vi "Key - MCListbox Read.vi"(8 "error in (no error)":errorcluster, 9 "New MulticolumnListbox Ref":refnum<vi>, 10 "Original MulticolumnListbox Ref":refnum<vi>, 11 "refnum":T1) -> (0 "error out":errorcluster, 2 "size(s)":i32[](array[numeric]), 3 "Refnum out":T1, 5 "Column Header Strings[]":string[](array[string]))   [LabVIEW 2013]
uses:
  <vilib>/Utility/config.llb/Config Data RefNum.ctl
  <vilib>/Utility/config.llb/Read Key (String).vi
  <vilib>/Utility/config.llb/NI_LVConfig.lvlib
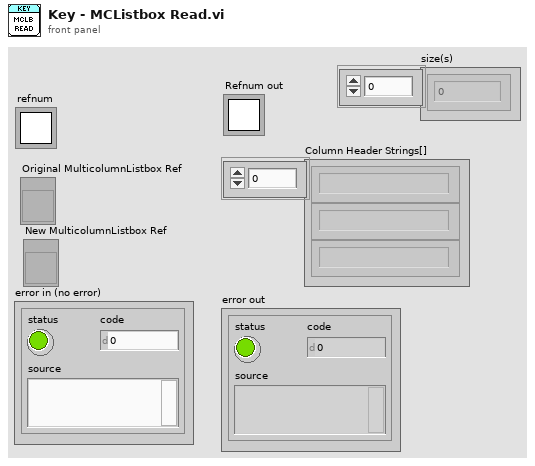
[diagram p1: front panel]
types:
  T1 = typedef "NI_LVConfig.lvlib/Config Data RefNum.ctl" = refnum<k1>
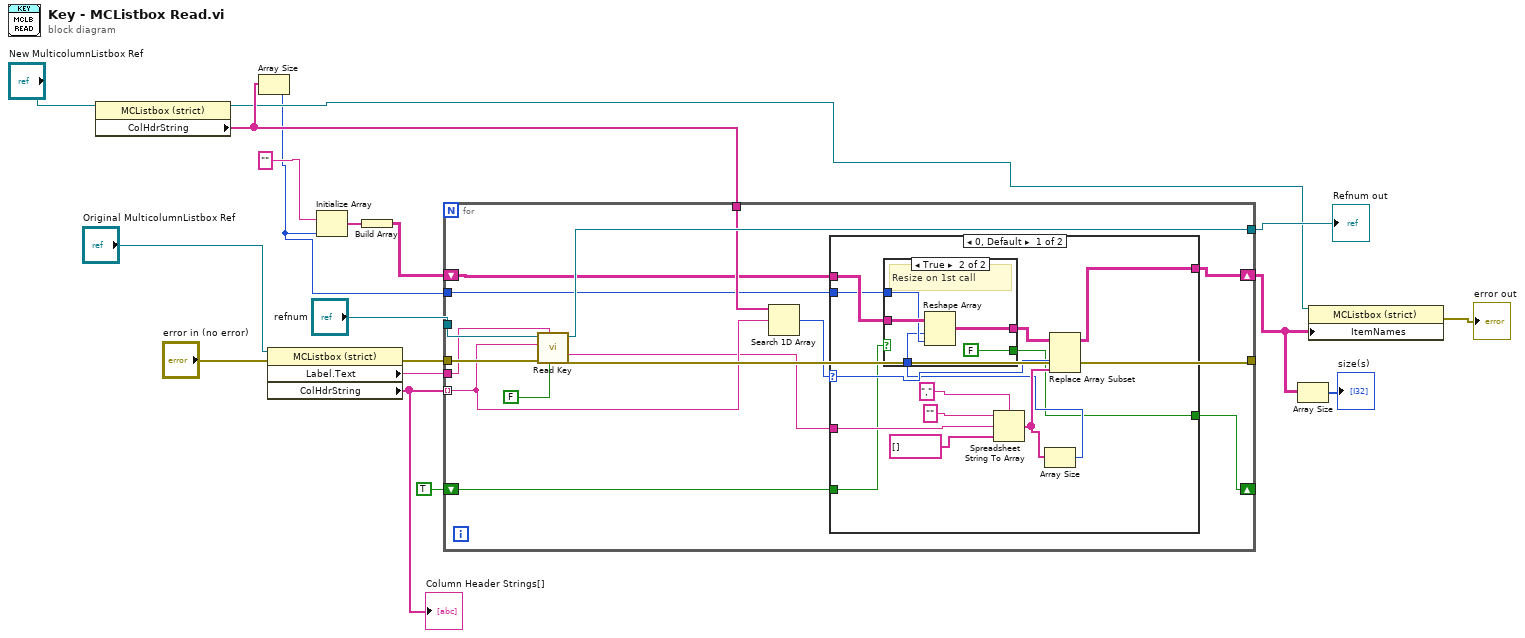
[diagram p0: block diagram]
diagram:
  n1 = property on="Property Node" class="MCListbox (strict)"(reference="New MulticolumnListbox Ref") -> (reference out=w10:refnum<vi>, "ColHdrString"=w11:string[])  [unwired: 1 in, 1 out]
  n2 = Array Size(array=w11) -> (size(s)=w5:i32)
  n3 = property on="Property Node" class="MCListbox (strict)"(reference="Original MulticolumnListbox Ref", error in="error in (no error)") -> (error out=w18:errorcluster, "Label.Text"=w13:string, "ColHdrString"=w4:string[])  [unwired: 1 out]
  "Column Header Strings[]" <- w4
  n4 = Initialize Array("" ("element"), w5) -> (w7:string[])
  n5 = Build Array(w7) -> (w6:string[][])
  n6 = for {
    tunnel: w18 -> [w33]
    tunnel: [w32] -> _
    tunnel: [w31] -> w16
    tunnel: "refnum" -> [w29]
    tunnel: w13 -> [w28]
    tunnel: w4 -> [w26] mode=indexing
    tunnel: w11 -> [w27]
    shift-right: [w23] -> w3
    shift-left: w6 -> [w24]
    tunnel: w5 -> [w21]
    shift-right: [w19] -> _
    shift-left: TRUE -> [w20]
    n7 = call-poly <vilib>:"Read Key.vi"("read raw string? (F)"=FALSE, "section"=w28, "error in (no error)"=w33, "key"=w26, "refnum"=w29) -> ("error out"=w32:errorcluster, "value"=w22:string, "refnum out"=w31:T1)  [unwired: 3 in, 1 out]
    n8 = Search 1D Array(1D array=w27, element=w26) -> (index of element=w25:i32)  [unwired: 1 in]
    n9 = case shown="0, Default" w25 {
      selector: w25 -> [w46 _]
      tunnel: w24 -> [w40 w55]
      tunnel: [w41 w55] -> w23
      tunnel: w22 -> [w42 _]
      tunnel: w21 -> [w38 _]
      tunnel: w20 -> [w35 w54]
      tunnel: [w34 w54] -> w19
      frame 0, Default {
        n10 = Spreadsheet String To Array(delimiter (Tab)=",", format string="", spreadsheet string=w42, array type (2D Dbl)=string[] []) -> (array=w37:string[])
        n11 = Array Size(array=w37) -> (size(s)=w36:i32)
        n12 = case shown="True" w35 {
          selector: w35 -> [w47 _]
          tunnel: w40 -> [w48 w53]
          tunnel: [w48 w52] -> w39
          tunnel: w38 -> [_ w51]
          tunnel: w36 -> [_ w50]
          tunnel: [w47 FALSE] -> w34
          frame False {
            # "Resized already"
          }
          frame True {
            # "Resize on 1st call"
            n13 = Reshape Array(w53, w50, w51) -> (w52:string[][])
          }
        }
        n14 = Replace Array Subset(array=w39, new element=w37, index (col)=w46) -> (w41:string[][])  [unwired: 1 in]
      }
      frame -1 {
      }
    }
  }
  "Refnum out" <- w16
  n15 = Array Size(array=w3) -> (size(s)=→"size(s)":i32[])
  n16 = property on="Property Node" class="MCListbox (strict)"(reference=w10, "ItemNames"=w3) -> (error out=→"error out":errorcluster)  [unwired: 1 in, 1 out]
